vi "Set String.vi"(5 "use temporary file? (F)":bool, 8 "error in":errorcluster, 9 "value":string, 10 "variable name":string, 11 "GOLPI ref. in":T1={"pipe handle"={"lv_proc.dll file path"=path "", "process instance handle"=[], "debug mode"=FALSE, "debug data"=[]}, "fast read timeout [ms]"=500, "fast read settle time [ms]"=10, "fast read to multiple [ms]"=1, "max elements per input line"=100, "slow read timeout [ms]"=5000, "stdin double format specifier"="%_16e", "max elements per stdout output column"=100, "console mode bitstream"=FALSE, "bitstream first read timeout [ms]"=1000, "bitstream read timeout [ms]"=50, "struct transfer possible"=FALSE, "matlab mode"=FALSE, "var pipe write timeout [ms]"=5000, "variable pipe mode"=FALSE, "variable pipe buffer size [Bytes]"=10000000, "variable pipe block size [Bytes]"=1000000} {"variable pipe block size [Bytes]" format="%.0p"; "variable pipe buffer size [Bytes]" format="%.0p"}) -> (0 "error out":errorcluster, 3 "GOLPI ref. out":T1={"pipe handle"={"lv_proc.dll file path"=path "", "process instance handle"=[], "debug mode"=FALSE, "debug data"=[]}, "fast read timeout [ms]"=500, "fast read settle time [ms]"=10, "fast read to multiple [ms]"=1, "max elements per input line"=100, "slow read timeout [ms]"=5000, "stdin double format specifier"="%_16e", "max elements per stdout output column"=100, "console mode bitstream"=FALSE, "bitstream first read timeout [ms]"=1000, "bitstream read timeout [ms]"=50, "struct transfer possible"=FALSE, "matlab mode"=FALSE, "var pipe write timeout [ms]"=5000, "variable pipe mode"=FALSE, "variable pipe buffer size [Bytes]"=10000000, "variable pipe block size [Bytes]"=1000000} {"variable pipe block size [Bytes]" format="%.0p"; "variable pipe buffer size [Bytes]" format="%.0p"})   [LabVIEW 2020, in "GOLPI library.lvlib"]
doc: "Part of polymorph Set Variable.vi"
uses:
  GOLPI library.lvlib
  Public/GOLPI reference Type Def.ctl
  LV Process source distribution/Pipe Handle.ctl
  LV Process source distribution/LV Process library.lvlib
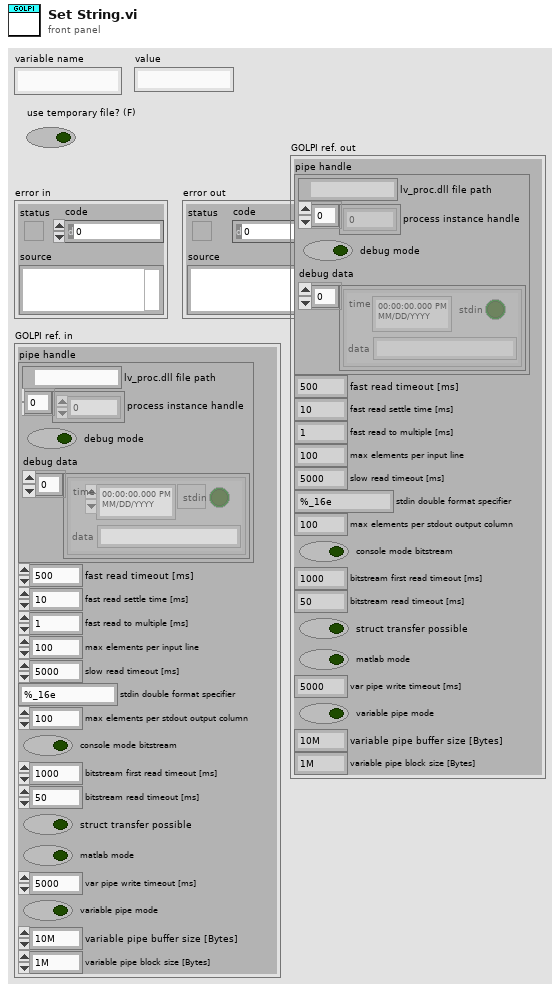
[diagram p1: front panel]
types:
  T1 = typedef "GOLPI library.lvlib/GOLPI reference Type Def.ctl" = cluster{"pipe handle":T2, "fast read timeout [ms]":u32, "fast read settle time [ms]":u32, "fast read to multiple [ms]":u32, "max elements per input line":u32, "slow read timeout [ms]":u32, "stdin double format specifier":string, "max elements per stdout output column":u32, "console mode bitstream":bool, "bitstream first read timeout [ms]":u32, "bitstream read timeout [ms]":u32, "struct transfer possible":bool, "matlab mode":bool, "var pipe write timeout [ms]":u32, "variable pipe mode":bool, "variable pipe buffer size [Bytes]":u32, "variable pipe block size [Bytes]":u32}
  T2 = typedef "LV Process library.lvlib/Pipe Handle.ctl" = cluster{"lv_proc.dll file path":path, "process instance handle":u32[], "debug mode":bool, "debug data":cluster{"time":timestamp, "stdin":bool, "data":string}[]}
  T3 = typedef "GOLPI library.lvlib/Transfer Mode.ctl" = enum16{"Matlab", "stdio", "temp file", "bitstream", "pipe"}
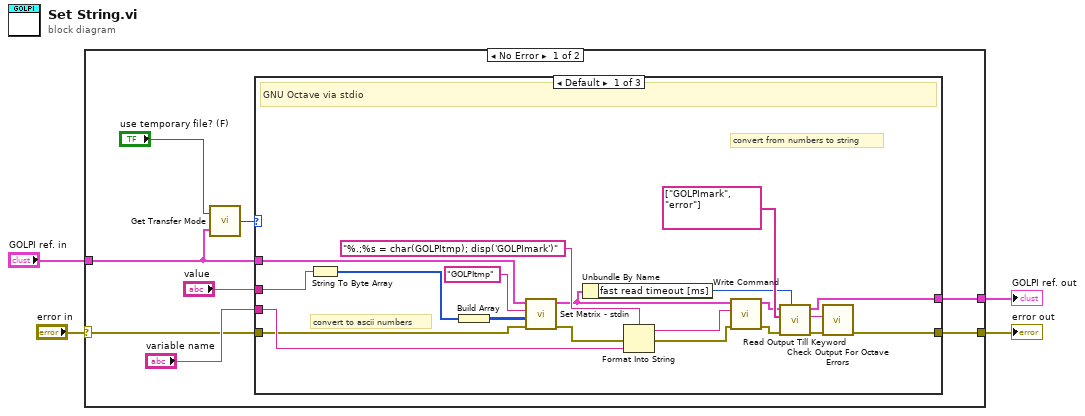
[diagram p0: block diagram]
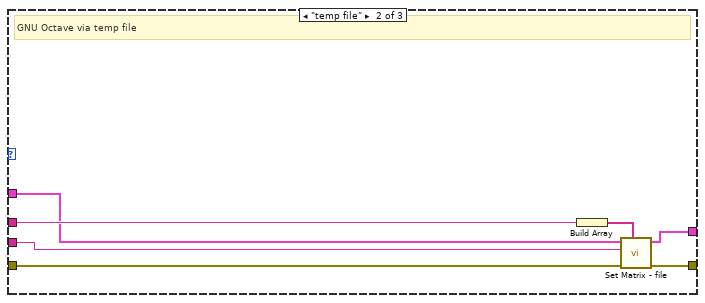
[diagram p2: hidden frame]
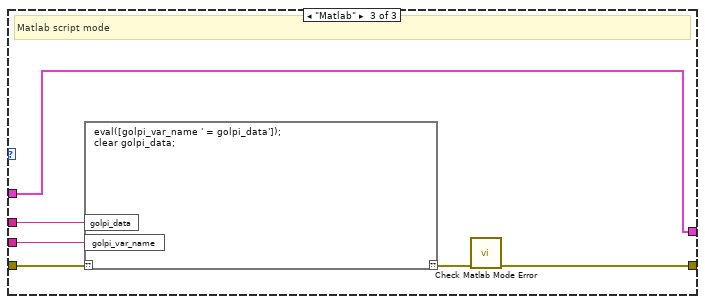
[diagram p3: hidden frame]
diagram:
  n1 = case shown="No Error" "error in" {
    selector: "error in" -> [w8 w47]
    tunnel: [w12 w47] -> w4
    tunnel: "GOLPI ref. in" -> [w6 w46]
    tunnel: [w11 w46] -> w1
    frame No Error {
      n2 = call "Get Transfer Mode.vi"("GOLPI ref."=w6, "use temporary file? (F)"="use temporary file? (F)") -> ("mode"=w7:T3)
      n3 = case shown="Default" w7 {
        tunnel: [w32 w39 w40] -> w12
        tunnel: [w31 w38 w44] -> w11
        tunnel: "variable name" -> [w30 w37 w42]
        tunnel: "value" -> [w29 w36 w43]
        tunnel: w8 -> [w28 w35 w45]
        tunnel: w6 -> [w27 w34 w44]
        frame Default {
          # "convert from numbers to string"
          # "convert to ascii numbers"
          # "GNU Octave via stdio"
          n4 = String To Byte Array(string=w29) -> (unsigned byte array=w17:u8[])
          n5 = Build Array(w17) -> (w16:u8[][])
          n6 = call "Set Matrix - stdin.vi"("error in"=w28, "value"=w16, "variable name"="GOLPItmp", "GOLPI ref. in"=w27) -> ("error out"=w14:errorcluster, "GOLPI ref. out"=w13:T1)  [unwired: 6 in]
          n7 = Unbundle By Name(w13) -> ("fast read timeout [ms]"=w18:u32)
          n8 = Format Into String(format string="%.;%s = char(GOLPItmp); disp('GOLPImark')", error in=w14, w30) -> (resulting string=w24:string, error out=w25:errorcluster)  [unwired: 1 in]
          n9 = call "Write Command.vi"("error in"=w25, "command"=w24, "GOLPI ref. in"=w13) -> ("error out"=w23:errorcluster, "GOLPI ref. out"=w20:T1)  [unwired: 7 in]
          n10 = call "Read Output Till Keyword.vi"("timeout [ms]"=w18, "error in"=w23, "keywords"=string[] ["GOLPImark", "error"], "GOLPI ref. in"=w20) -> ("error out"=w22:errorcluster, "read buffer"=w19:string, "GOLPI ref. out"=w31:T1)  [unwired: 4 in, 1 out]
          n11 = call "Check Output For Octave Errors.vi"("error in"=w22, "read buffer"=w19) -> ("error out"=w32:errorcluster)  [unwired: 9 in]
        }
        frame "temp file" {
          # "GNU Octave via temp file"
          n12 = Build Array(w36) -> (w33:string[])
          n13 = call "Set Matrix - file.vi"("string array"=w33, "error in (no error)"=w35, "variable name"=w37, "GOLPI ref. in"=w34) -> ("error out"=w39:errorcluster, "GOLPI ref. out"=w38:T1)  [unwired: 6 in]
        }
        frame "Matlab" {
          # "Matlab script mode"
          n14 = script code="eval([golpi_var_name ' = golpi_data']);\nclear golpi_data;"("??"=w45, "golpi_var_name"=w42, "golpi_data"=w43) -> ("??"=w41:errorcluster)
          n15 = call "Check Matlab Mode Error.vi"("error in"=w41) -> ("error out"=w40:errorcluster)  [unwired: 10 in]
        }
      }
    }
    frame Error {
    }
  }
  "error out" <- w4
  "GOLPI ref. out" <- w1
